vi "1A_ArbTriggeredOn.vi"(5 "Frequency (Hz)":dbl=40000.0, 7 "Amplitude (Vpp)":dbl=3.2, 11 "error in":errorcluster) -> (15 "error out":errorcluster)   [LabVIEW 2010]
uses:
  <instrlib>/Agilent 33XXX Series/Agilent 33XXX Series.lvlib
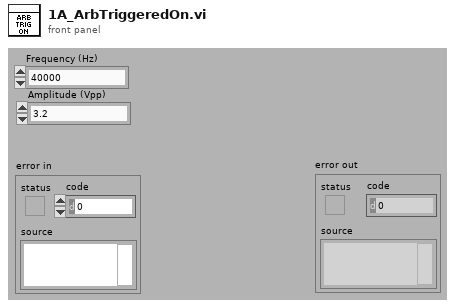
[diagram p1: front panel]
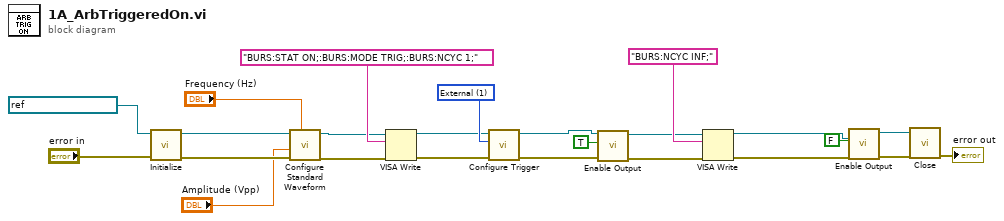
[diagram p0: block diagram]
diagram:
  w20 = u16 1 items=["Internal", "External", "Software (bus)"] ("Trigger Source (0: Internal)")
  n1 = call <instrlib>:"Initialize.vi"("error in (no error)"="error in", "VISA resource name"=refnum<visa-resource-name> "GPIB0::7::INSTR") -> ("error out"=w22:errorcluster, "VISA resource name out"=w21:refnum<visa-resource-name>)  [unwired: 8 in]
  n2 = call <instrlib>:"Configure Standard Waveform.vi"("Frequency (1000 Hz)"="Frequency (Hz)", "error in (no error)"=w22, "Amplitude (1)"="Amplitude (Vpp)", "VISA resource name"=w21) -> ("error out"=w12:errorcluster, "VISA resource name out"=w13:refnum<visa-resource-name>)  [unwired: 6 in]
  n3 = VISA Write(VISA resource name=w13, write buffer="BURS:STAT ON;:BURS:MODE TRIG;:BURS:NCYC 1;", error in (no error)=w12) -> (VISA resource name out=w16:refnum<visa-resource-name>, error out=w15:errorcluster)  [unwired: 1 out]
  n4 = call <instrlib>:"Configure Trigger.vi"("error in (no error)"=w15, "Trigger Source (0: Internal)"=w20, "VISA resource name"=w16) -> ("error out"=w6:errorcluster, "VISA resource name out"=w7:refnum<visa-resource-name>)  [unwired: 7 in]
  n5 = call <instrlib>:"Enable Output.vi"("error in (no error)"=w6, "Enable Output  (T: Enable)"=TRUE, "VISA resource name"=w7) -> ("error out"=w4:errorcluster, "VISA resource name out"=w5:refnum<visa-resource-name>)  [unwired: 7 in]
  n6 = VISA Write(VISA resource name=w5, write buffer="BURS:NCYC INF;", error in (no error)=w4) -> (VISA resource name out=w10:refnum<visa-resource-name>, error out=w9:errorcluster)  [unwired: 1 out]
  n7 = call <instrlib>:"Enable Output.vi"("error in (no error)"=w9, "Enable Output  (T: Enable)"=FALSE, "VISA resource name"=w10) -> ("error out"=w18:errorcluster, "VISA resource name out"=w19:refnum<visa-resource-name>)  [unwired: 7 in]
  n8 = call <instrlib>:"Close.vi"("error in (no error)"=w18, "VISA resource name"=w19) -> ("error out"=→"error out":errorcluster)  [unwired: 9 in]
